vi "GT Get Ext Ad Value.vi"(7 "pValue":u16[](array[numeric]), 8 "error in (no error)":errorcluster caption="错误输入（无错误）", 9 "chn":i16, 10 "mdl":i16, 11 "cardNum":i16) -> (0 "error out":errorcluster caption="错误输出", 3 "function return":i16, 5 "pValue out":u16[](array[numeric]))   [LabVIEW 2020, in "gts.lvlib"]
doc: "GT_API GT_GetExtAdValue(short cardNum,short mdl,short chn,unsigned short *pValue);"
uses:
  gts.lvlib
  dll/32bit/multi_card/gts.dll
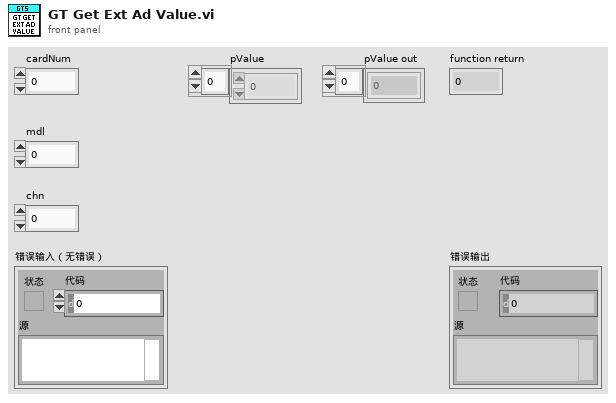
[diagram p1: front panel]
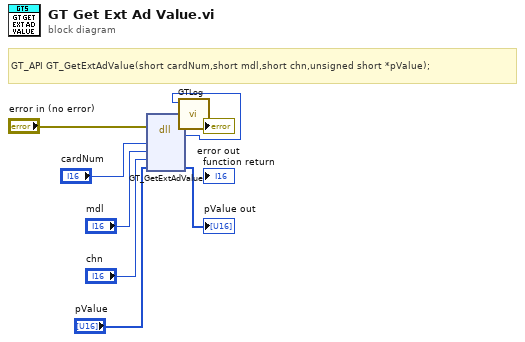
[diagram p0: block diagram]
diagram:
  # "GT_API GT_GetExtAdValue(short cardNum,short mdl,short chn,unsigned short *pValue);"
  n1 = dll-call lib="C:/1228/dll/32bit/multi_card/gts.dll" fn="GT_GetExtAdValue"(error in="error in (no error)", "cardNum"="cardNum", "mdl"="mdl", "chn"="chn", "pValue"="pValue") -> (error out=w3:errorcluster, "返回类型"=w1:i16, "pValue"=→"pValue out":u16[])  [unwired: 5 in, 1 out]
  n2 = call "GTLog.vi"("error in (no error)"=w3, "Numeric"=w1) -> ("error out"=→"error out":errorcluster)  [unwired: 9 in]
